vi "UDP Read Peek Test.vi"() -> ()   [LabVIEW 2014, in "ESP8266 WiFi Wrapper.lvlib"]
uses:
  <vilib>/Aledyne-TSXperts/Arduino Compatible Compiler for LabVIEW/addons/ESP8266 WiFi Wrapper/ESP8266 WiFi Wrapper.lvlib
panel:
  out "Next byte":u8
  out "Read byte":u8
  out "Error Out":errorcluster
  in  "Error In":errorcluster
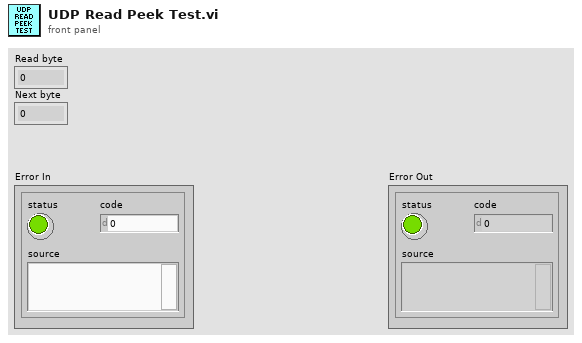
[diagram p1: front panel]
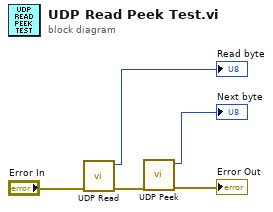
[diagram p0: block diagram]
diagram:
  n1 = call <vilib>:"UDP Read.vi"("Error In"="Error In") -> ("Error Out"=w3:errorcluster, "Read byte"=→"Read byte":u8)  [unwired: 9 in]
  n2 = call <vilib>:"UDP Peek.vi"("Error In"=w3) -> ("Error Out"=→"Error Out":errorcluster, "Next byte"=→"Next byte":u8)  [unwired: 9 in]
